vi "Snap4.vi"(1 "x":dbl) -> (0 "x out":dbl)   [LabVIEW 2024]
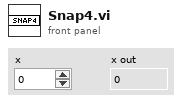
[diagram p1: front panel]
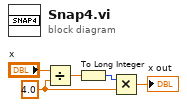
[diagram p0: block diagram]
diagram:
  w3 = 4.0 ("y")
  n1 = Divide(x="x", y=w3) -> (x/y=w5:dbl)
  n2 = To Long Integer(number=w5) -> (32bit integer=w4:i32)
  n3 = Multiply(x=w4, y=w3) -> (x*y=→"x out":dbl)
